vi "test_LocationFGV_ReresolveLocation_LocationResolved.vi"(8 "error in":errorcluster) -> (0 "error out":errorcluster, 2 "result":string, 3 "pass":bool)   [LabVIEW 2020, in "MeasurementServerTests.lvlib" / "gRPC Utilities Tests.lvlib"]
uses:
  gRPC Utilities Tests.lvlib
  Fake Location Action.ctl
  Runtime/MeasurementLink Discovery/TypeDefs/Service Location FGV Action.ctl
  Runtime/MeasurementLink Discovery/MeasurementLink Discovery.lvlib
  Runtime/MeasurementLink Discovery Client/RPC Messages/ni_measurementlink_discovery_v1_ResolveServiceRequest.ctl
  Runtime/MeasurementLink Discovery Client/MeasurementLink Discovery Client.lvlib
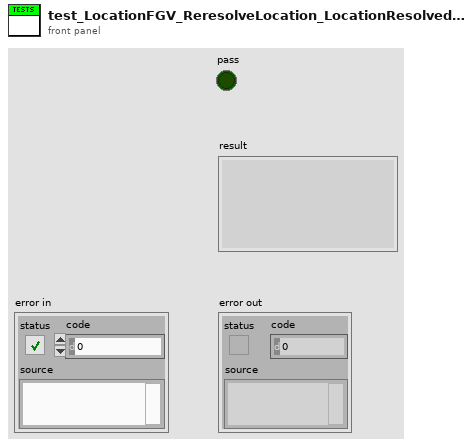
[diagram p1: front panel]
types:
  T1 = typedef "MeasurementLink Discovery Client.lvlib/ni_measurementlink_discovery_v1_ResolveServiceRequest.ctl" = cluster{"provided_interface":string, "service_class":string}
  T2 = typedef "MeasurementLink Discovery.lvlib/Service Location FGV Action.ctl" = enum16{"Get Service Location", "Reresolve Service Location"}
  T3 = typedef "MeasurementServerTests.lvlib/gRPC Utilities Tests.lvlib/Fake Location Action.ctl" = enum16{"Generate New Location", "Reset", "Error on Next Call"}
  T4 = typedef "MeasurementLink Discovery Client.lvlib/ni_measurementlink_discovery_v1_ServiceLocation.ctl" = cluster{"location":string, "insecure_port":string, "ssl_authenticated_port":string}
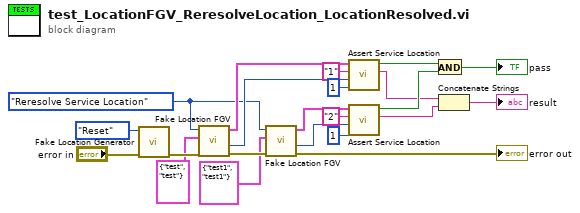
[diagram p0: block diagram]
diagram:
  w1 = Service_Location_FGV_Action."Reresolve Service Location" ("action")
  n1 = call "Fake Location Generator.vi"("error in"="error in", "action"=Fake_Location_Action."Reset") -> ("error out"=w21:errorcluster)  [unwired: 8 in, 1 out]
  n2 = call "Fake Location FGV.vi"("error in"=w21, "resolve service request"=T1 {"provided_interface"="test", "service_class"="test"}, "action"=w1) -> ("error out"=w18:errorcluster, "unique id out"=w15:u64, "service location"=w16:T4)  [unwired: 6 in]
  n3 = call "Fake Location FGV.vi"("error in"=w18, "resolve service request"=T1 {"provided_interface"="test1", "service_class"="test1"}, "action"=w1) -> ("error out"=→"error out":errorcluster, "unique id out"=w12:u64, "service location"=w14:T4)  [unwired: 6 in]
  n4 = call "Assert Service Location.vi"("expected unique id"=u64 1, "actual unique id"=w15, "expected service location port"="1", "actual service location"=w16) -> ("result"=w4:string, "pass"=w7:bool)  [unwired: 6 in]
  n5 = call "Assert Service Location.vi"("expected unique id"=u64 1, "actual unique id"=w12, "expected service location port"="2", "actual service location"=w14) -> ("result"=w3:string, "pass"=w6:bool)  [unwired: 6 in]
  n6 = And(x=w7, y=w6) -> (x .and. y?=→"pass":bool)
  n7 = Concatenate Strings(w4, w3) -> (→"result":string)
